vi "Strain initial.vi"(8 "error in":errorcluster caption="에러 입력", 10 "Sample Number":i32=100, 11 "Sampling rate":dbl=1000.0) -> (0 "error out":errorcluster caption="에러 출력", 3 "task out":refnum<k21> caption="태스크 출력")   [LabVIEW 2013]
uses:
  <vilib>/DAQmx/configure/timing.llb/DAQmx Timing (Sample Clock).vi
  <vilib>/DAQmx/create/channels.llb/DAQmx Create Channel (AI-Strain-Strain Gage).vi
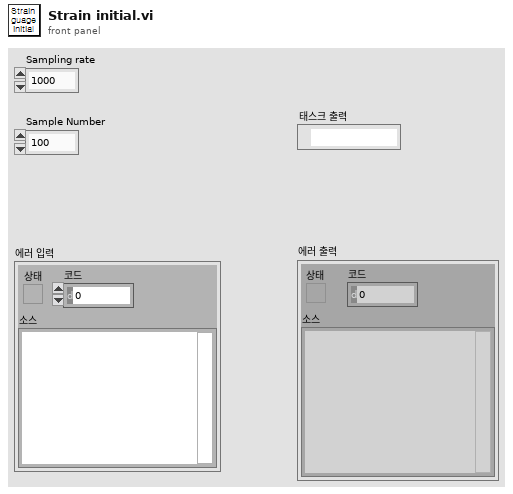
[diagram p1: front panel]
types:
  T1 = cluster{"gage factor":dbl, "nominal gage resistance":dbl, "poisson ratio":dbl}
  T2 = cluster{"strain configuration":i32, "lead wire resistance":dbl, "initial bridge voltage":dbl, "voltage excitation source":i32, "voltage excitation value":dbl}
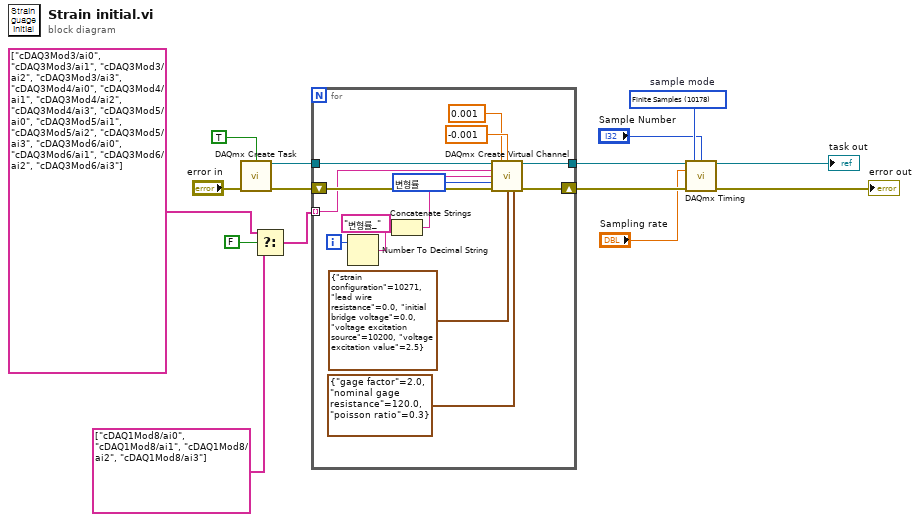
[diagram p0: block diagram]
diagram:
  w10 = 10178 items=["Finite Samples"=10178, "Continuous Samples"=10123, "Hardware Timed Single Point"=12522]  # sample mode
  n1 = call <vilib>:"DAQmx Create Task.vi"("auto cleanup"=TRUE, "error in"="error in") -> ("task out"=w13:refnum<k21>, "error out"=w15:errorcluster)  [unwired: 12 in]
  n2 = Select(t=tag[] ["cDAQ3Mod3/ai0", "cDAQ3Mod3/ai1", "cDAQ3Mod3/ai2", "cDAQ3Mod3/ai3", "cDAQ3Mod4/ai0", "cDAQ3Mod4/ai1", "cDAQ3Mod4/ai2", "cDAQ3Mod4/ai3", "cDAQ3Mod5/ai0", "cDAQ3Mod5/ai1", "cDAQ3Mod5/ai2", "cDAQ3Mod5/ai3", "cDAQ3Mod6/ai0", "cDAQ3Mod6/ai1", "cDAQ3Mod6/ai2", "cDAQ3Mod6/ai3"], s=FALSE, f=tag[] ["cDAQ1Mod8/ai0", "cDAQ1Mod8/ai1", "cDAQ1Mod8/ai2", "cDAQ1Mod8/ai3"]) -> (s? t:f=w4:tag[])
  n3 = for "For 루프" {
    tunnel: w13 -> [w29]
    tunnel: [w27] -> w11
    shift-right: [w26] -> w12
    shift-left: w15 -> [w28]
    tunnel: w4 -> [w19] mode=indexing
    i -> [w25]
    w18 = 10299 items=["변형률"=10299, "사용자 스케일로부터"=10065] ("units")
    n4 = Number To Decimal String(number=w25) -> (decimal integer string=w23:string)  [unwired: 1 in]
    n5 = Concatenate Strings("변형률_", w23) -> (w24:string)
    n6 = call-poly <vilib>:"DAQmx Create Virtual Channel.vi"("task in"=w29, "maximum value"=0.001, "minimum value"=-0.001, "physical channels"=w19, "name to assign"=w24, "units"=w18, "error in"=w28, "bridge information"=T2 {"strain configuration"=10271, "lead wire resistance"=0.0, "initial bridge voltage"=0.0, "voltage excitation source"=10200, "voltage excitation value"=2.5}, "strain gage information"=T1 {"gage factor"=2.0, "nominal gage resistance"=120.0, "poisson ratio"=0.3}) -> ("task out"=w27:refnum<k21>, "error out"=w26:errorcluster)  [unwired: 5 in]
  }
  n7 = call-poly <vilib>:"DAQmx Timing.vi"("task/channels in"=w11, "sample mode"=w10, "samples per channel"="Sample Number", "rate"="Sampling rate", "error in"=w12) -> ("task out"=→"task out":refnum<k21>, "error out"=→"error out":errorcluster)  [unwired: 9 in]
